vi "Run.vi"(8 "error in (no error)":errorcluster, 11 "Opctics in":refnum<class "Optics.lvclass">) -> (0 "error out":errorcluster, 3 "Optics out":refnum<class "Optics.lvclass">)   [LabVIEW 2018, in "Optics.lvclass"]
uses:
  Optics.lvclass
  Optics.lvclass/Optics.ctl
  Device.lvclass
  StateMachine/State Machine.lvclass
panel:
  out "on target 3":bool
  out "on target 2":bool
  out "on target":bool
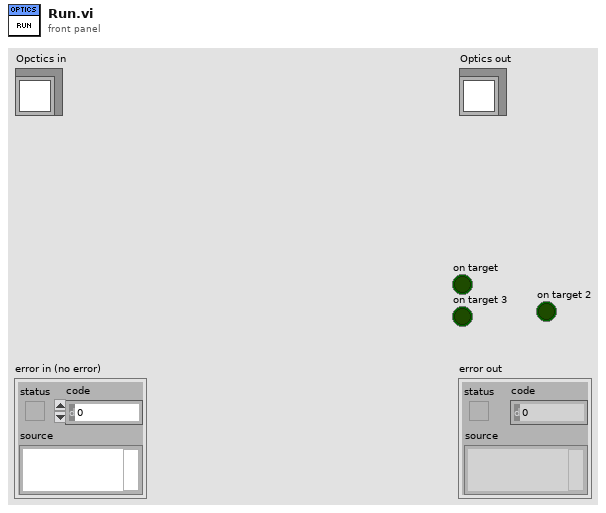
[diagram p1: front panel]
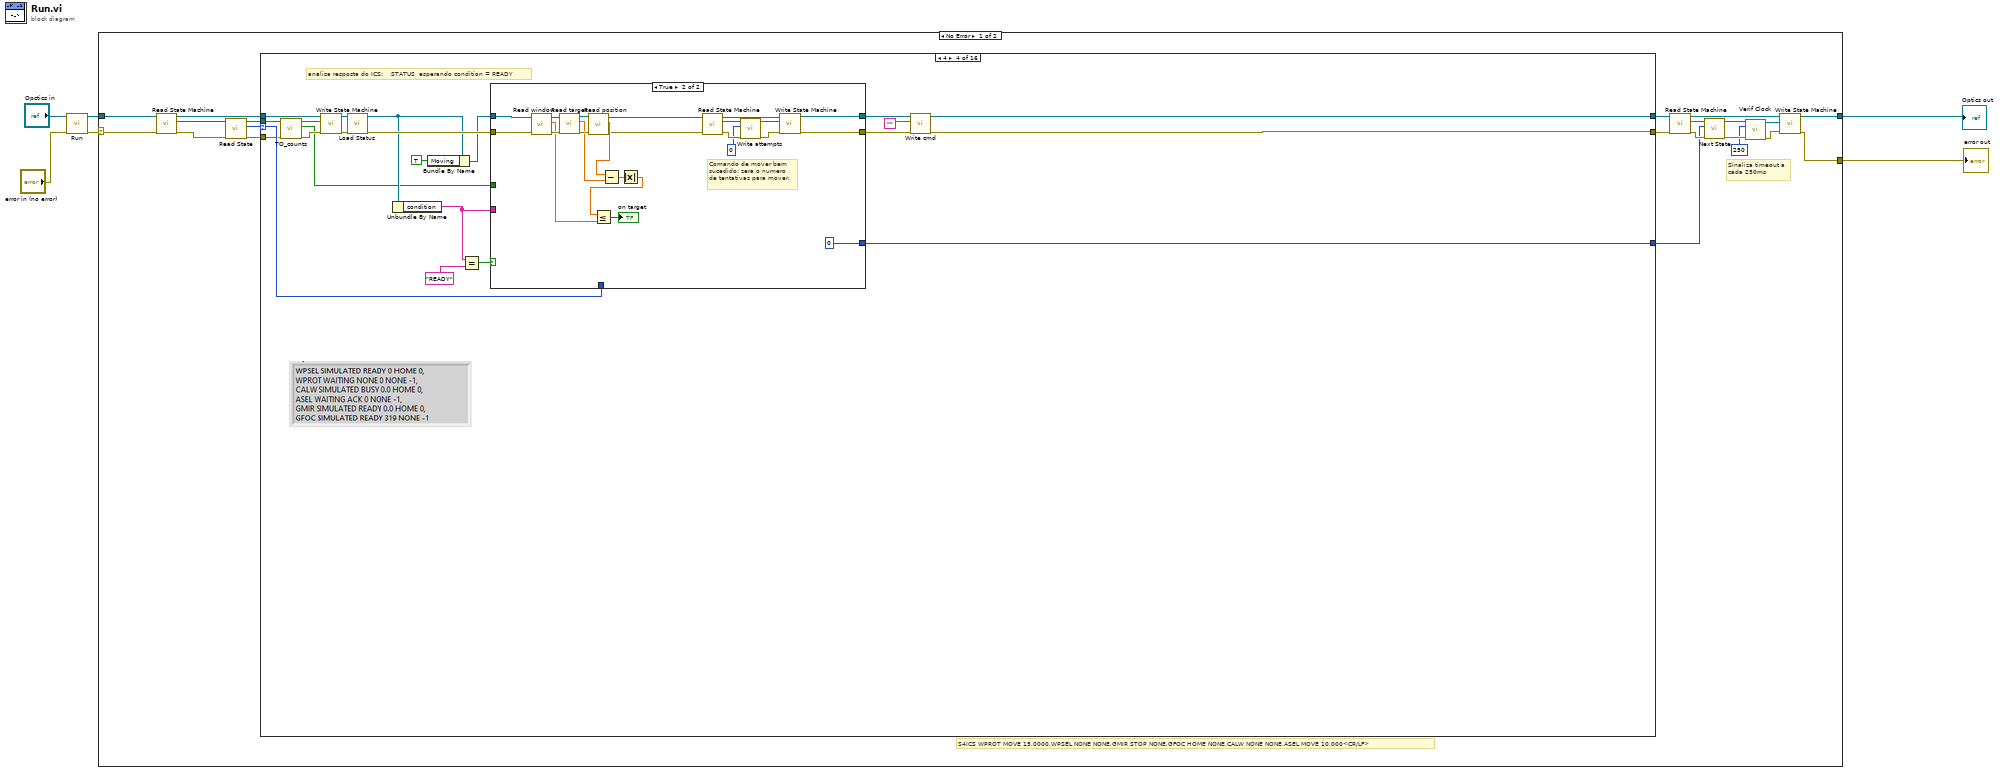
[diagram p0: block diagram]
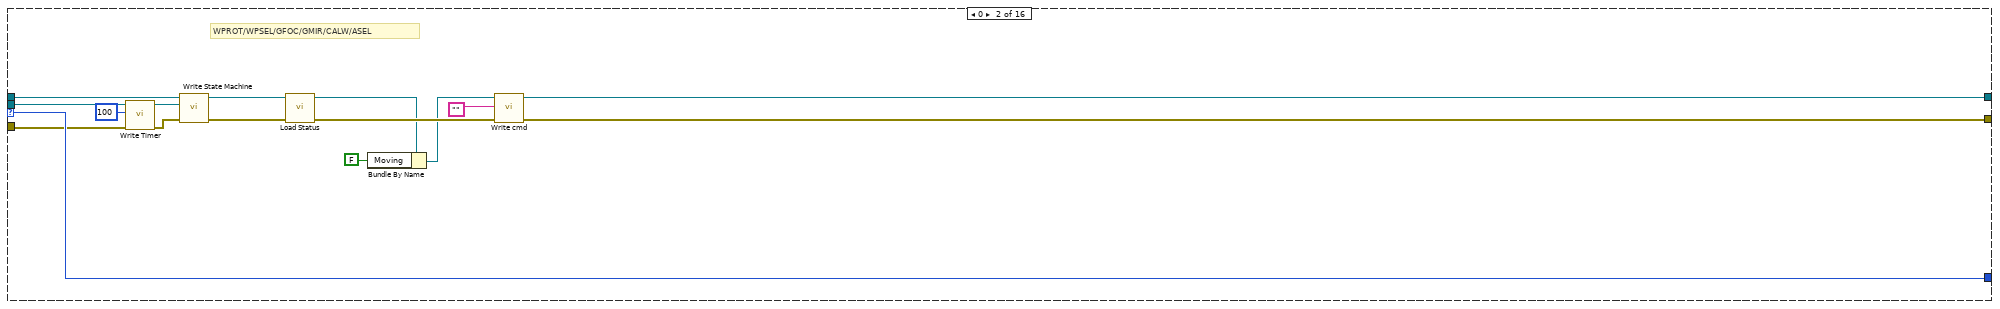
[diagram p3: hidden frame]
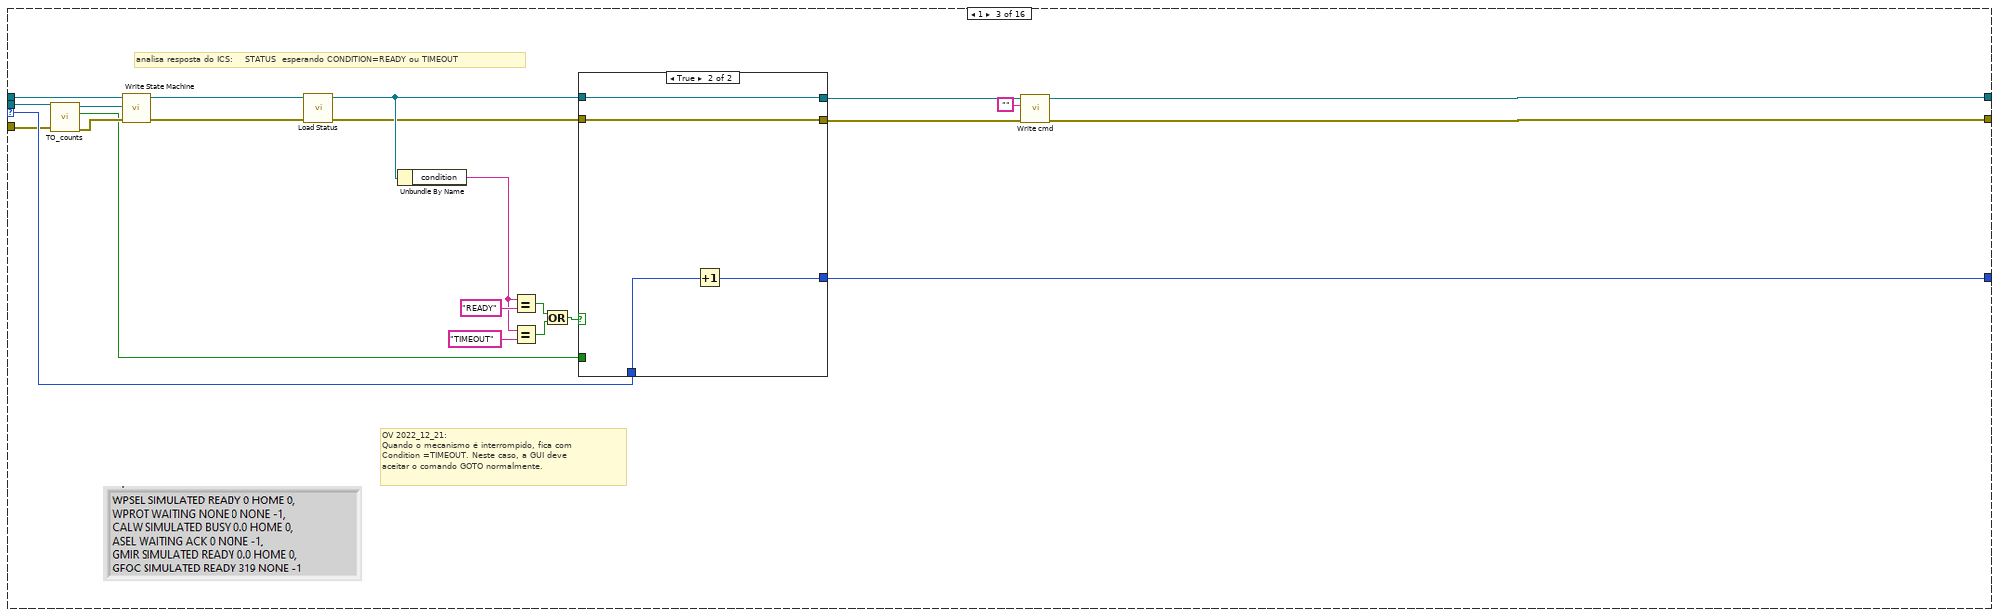
[diagram p4: hidden frame]
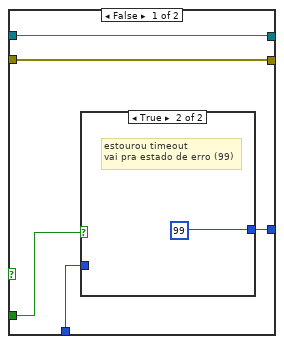
[diagram p5: hidden frame]
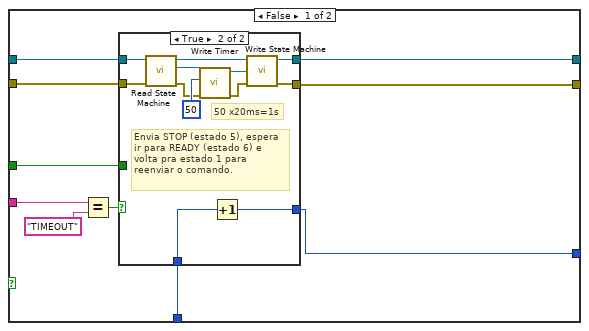
[diagram p7: hidden frame]
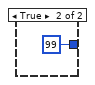
[diagram p9: hidden frame]
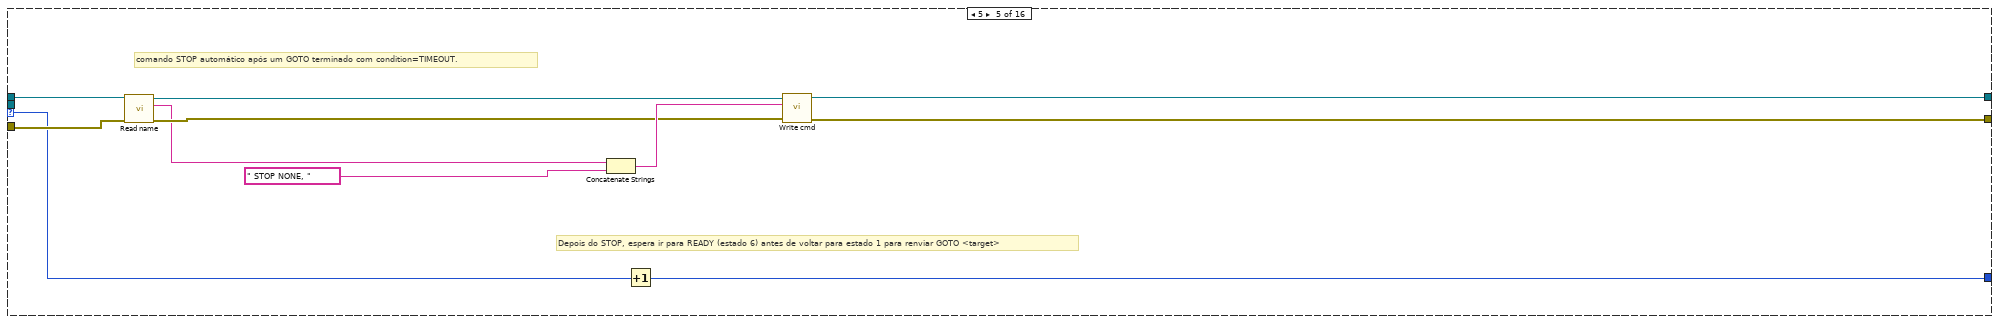
[diagram p10: hidden frame]
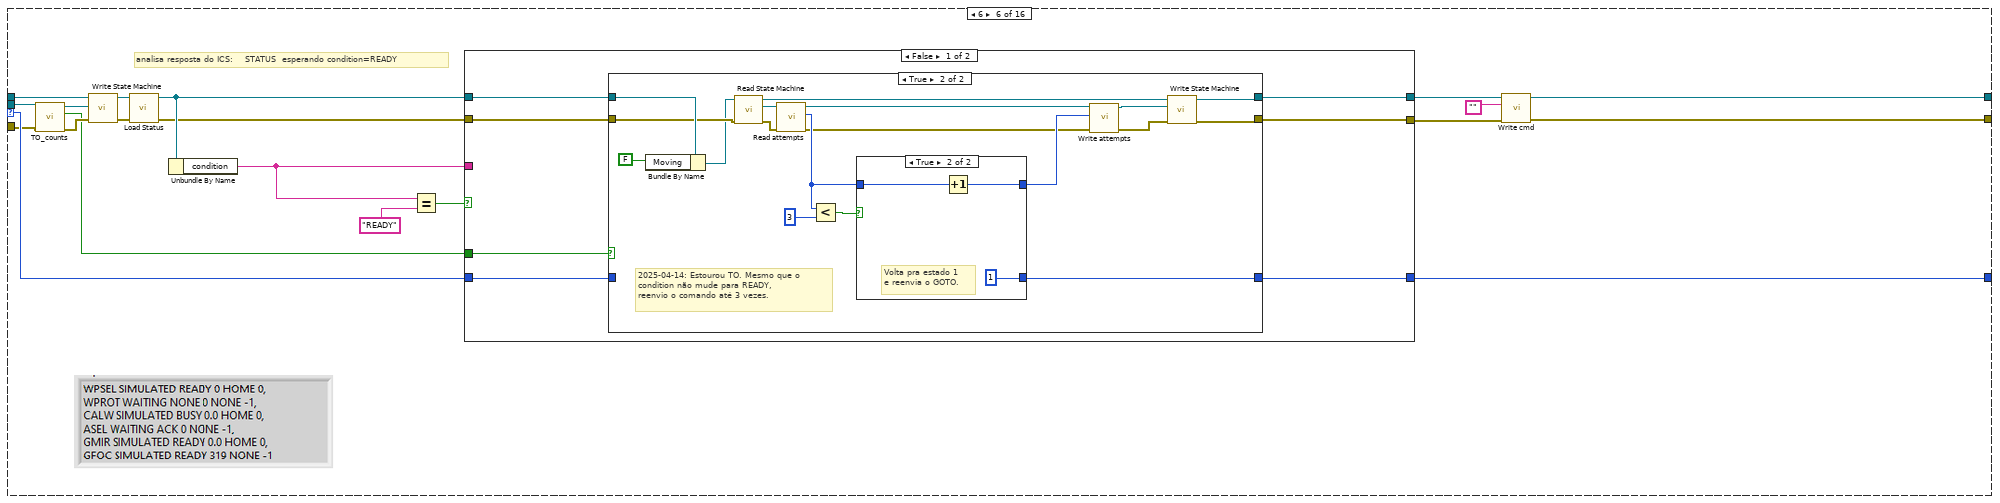
[diagram p11: hidden frame]
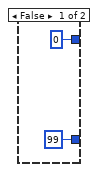
[diagram p13: hidden frame]
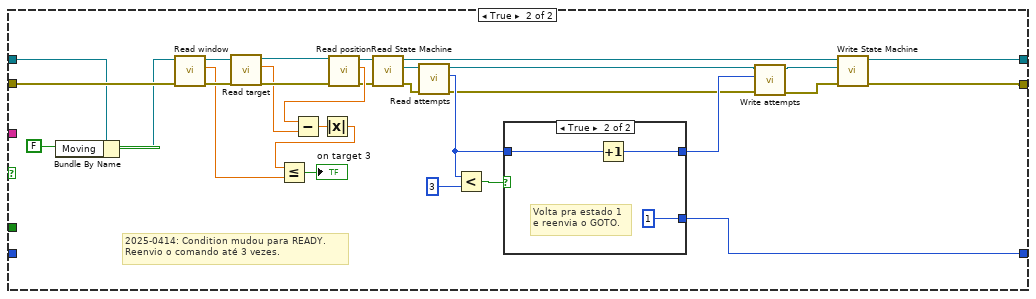
[diagram p14: hidden frame]
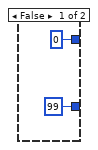
[diagram p15: hidden frame]
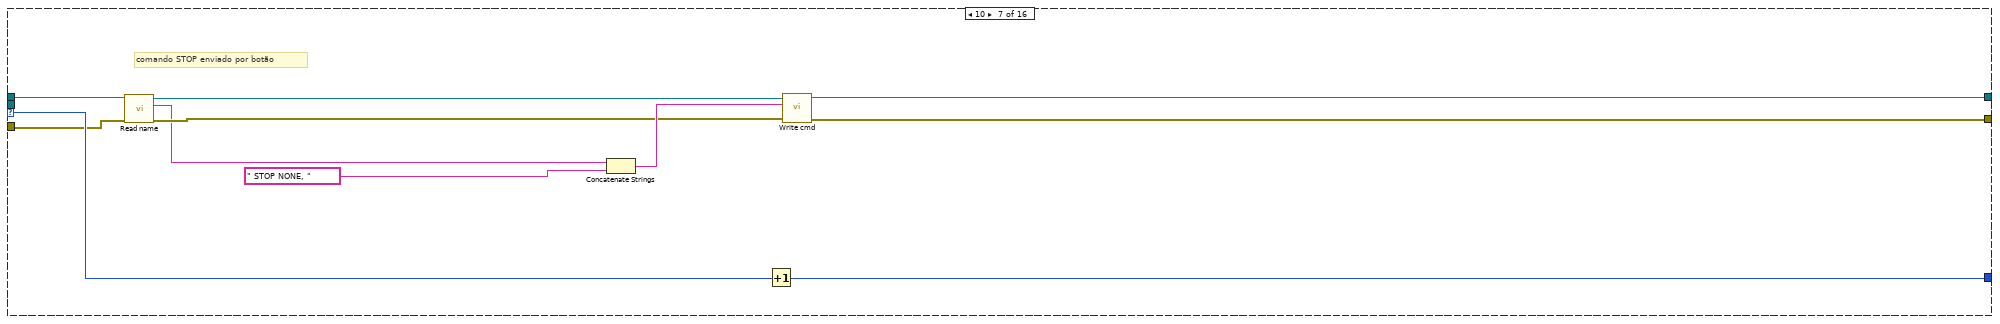
[diagram p16: hidden frame]
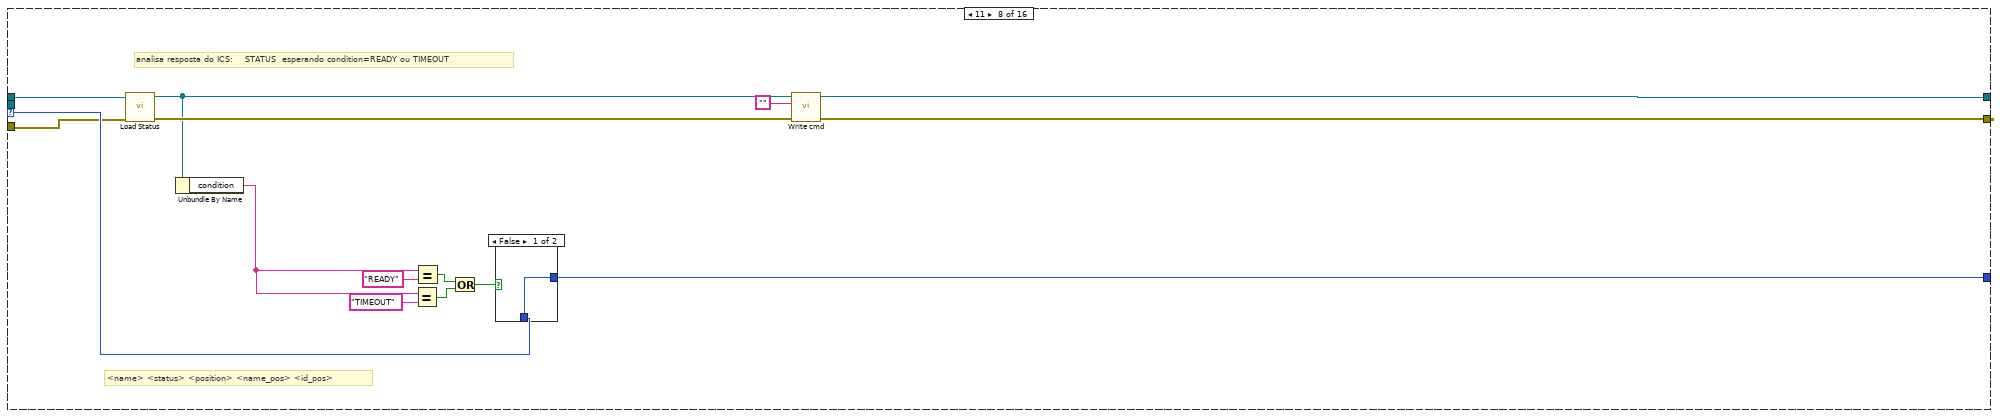
[diagram p17: hidden frame]
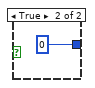
[diagram p18: hidden frame]
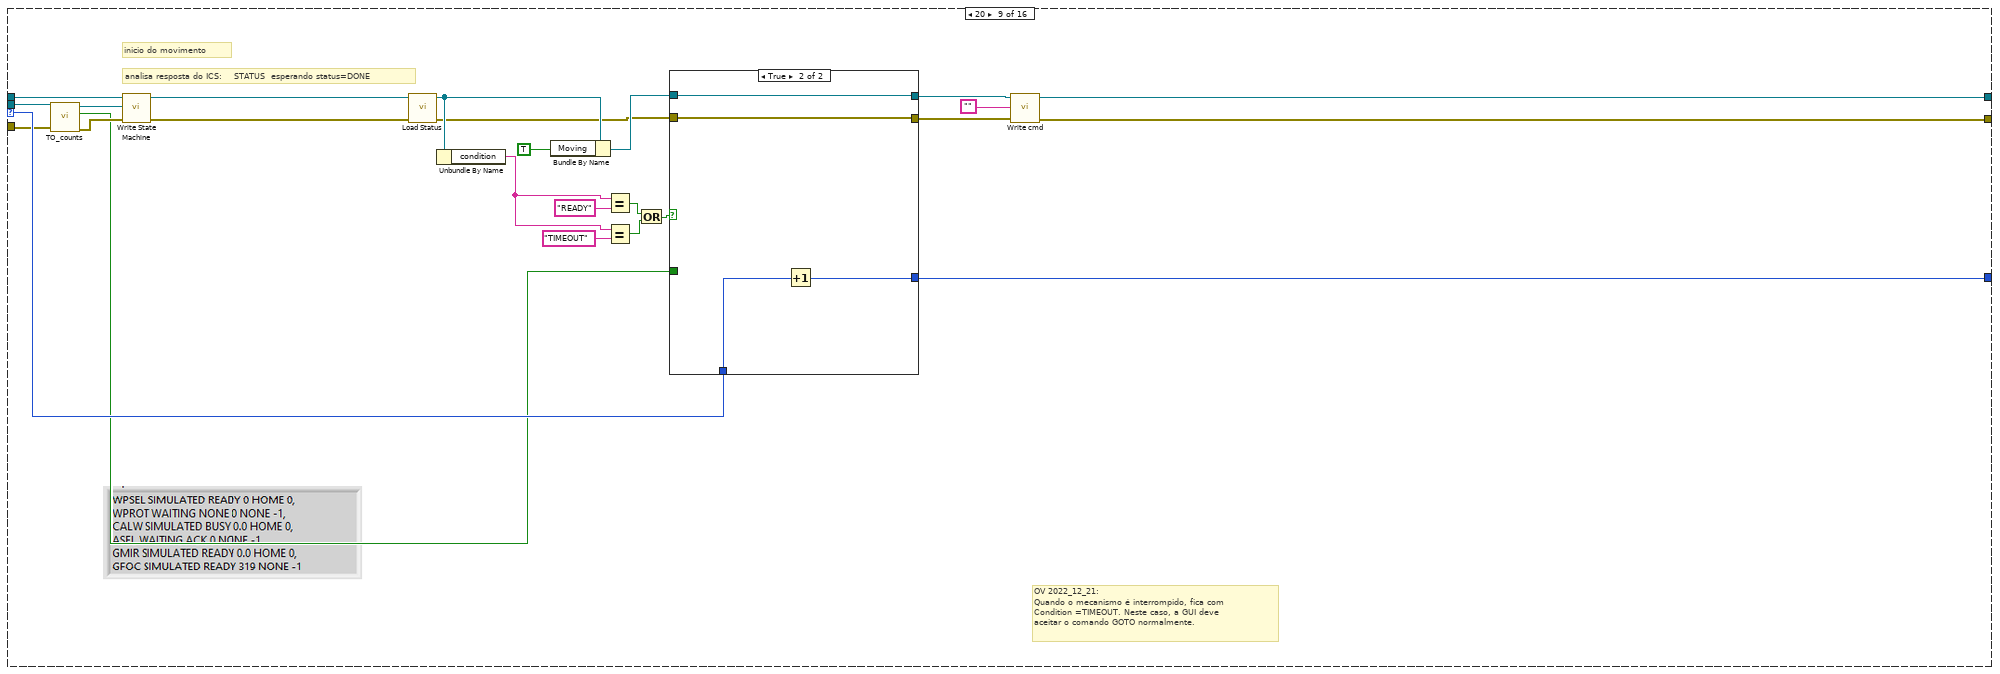
[diagram p19: hidden frame]
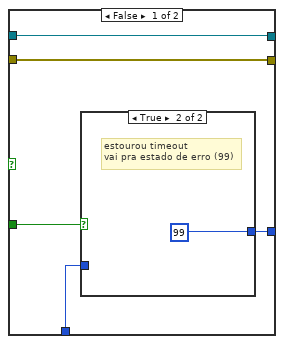
[diagram p20: hidden frame]
diagram:
  n1 = call-parent "Run.vi"("error in (no error)"="error in (no error)", "Device in"="Opctics in") -> ("error out"=w4:errorcluster, "Device out"=w3:refnum<class "Optics.lvclass">)  [unwired: 8 in]
  n2 = case shown="No Error" w4 {
    selector: w4 -> [w16 w465]
    tunnel: [w19 w465] -> w1
    tunnel: [w22 w464] -> w2
    tunnel: w3 -> [w17 w464]
    frame No Error {
      # "Sinaliza timeout a\ncada 250ms"
      # "S4ICS WPROT MOVE 15.0000,WPSEL NONE NONE,GMIR STOP NONE,GFOC HOME NONE,CALW NONE NONE,ASEL MOVE 10.000<CR/LF>"
      n3 = call-dynamic "Read State Machine.vi"("error in (no error)"=w16, "Device in"=w17) -> ("error out"=w15:errorcluster, "State Machine.lvclass"=w14:refnum<class "State Machine.lvclass">, "Device out"=w25:refnum<class "Optics.lvclass">)  [unwired: 7 in]
      n4 = call-dynamic "Read State.vi"("error in (no error)"=w15, "State Machine in"=w14) -> ("error out"=w26:errorcluster, "State"=w27:i32, "State Machine out"=w18:refnum<class "State Machine.lvclass">)  [unwired: 7 in]
      n5 = case shown="4" w27 {
        selector: w27 -> [w28 w43 w66 w99 w156 w182 w261 w279 w303 w331 w347 w381 w403 w422 w441 w461]
        tunnel: w26 -> [w29 w41 w62 w81 w159 w171 w256 w268 w299 w322 w340 w375 w395 w416 w434 w456]
        tunnel: [w29 w45 w68 w101 w164 w184 w263 w276 w305 w328 w349 w384 w400 w420 w438 w462] -> w8
        tunnel: w25 -> [w30 w42 w65 w85 w161 w169 w258 w269 w302 w323 w339 w374 w399 w423 w437 w457]
        tunnel: [w30 w46 w69 w102 w165 w185 w264 w277 w306 w329 w350 w385 w401 w421 w439 w463] -> w7
        tunnel: [w28 w43 w67 w100 w155 w183 w262 w278 w304 w330 w348 w382 w402 w419 w440 w461] -> w20
        tunnel: w18 -> [_ w39 w64 w86 _ w170 _ _ w301 _ _ w376 w397 w418 w436 _]
        frame Default {
        }
        frame 0 {
          # "WPROT/WPSEL/GFOC/GMIR/CALW/ASEL"
          n6 = call-dynamic "Write Timer.vi"("error in (no error)"=w41, "Timer"=u32 100, "State Machine in"=w39) -> ("error out"=w40:errorcluster, "State Machine out"=w38:refnum<class "State Machine.lvclass">)  [unwired: 7 in]
          n7 = call-dynamic "Write State Machine.vi"("error in (no error)"=w40, "State Machine.lvclass"=w38, "Device in"=w42) -> ("error out"=w35:errorcluster, "Device out"=w36:refnum<class "Optics.lvclass">)  [unwired: 7 in]
          n8 = call-dynamic "Load Status.vi"("error in (no error)"=w35, "Optics in"=w36) -> ("error out"=w34:errorcluster, "Optics out"=w33:refnum<class "Optics.lvclass">)  [unwired: 8 in]
          n9 = Bundle By Name(cluster=w33, "Moving"=FALSE) -> (w31:refnum<class "Optics.lvclass">)
          n10 = call-dynamic "Write cmd.vi"("error in (no error)"=w34, "cmd"="", "Device in"=w31) -> ("error out"=w45:errorcluster, "Device out"=w46:refnum<class "Optics.lvclass">)  [unwired: 7 in]
        }
        frame 1 {
          # "OV 2022_12_21:\nQuando o mecanismo é interrompido, fica com\nCondition =TIMEOUT. Neste caso, a GUI deve\naceitar o comando GOTO normalmente."
          # "analisa resposta do ICS:    STATUS  esperando CONDITION=READY ou TIMEOUT"
          n11 = call-dynamic "TO_counts.vi"("error in (no error)"=w62, "State Machine in"=w64) -> ("error out"=w61:errorcluster, "timer zero"=w60:bool, "State Machine out"=w63:refnum<class "State Machine.lvclass">)  [unwired: 7 in]
          n12 = call-dynamic "Write State Machine.vi"("error in (no error)"=w61, "State Machine.lvclass"=w63, "Device in"=w65) -> ("error out"=w50:errorcluster, "Device out"=w51:refnum<class "Optics.lvclass">)  [unwired: 7 in]
          n13 = call-dynamic "Load Status.vi"("error in (no error)"=w50, "Optics in"=w51) -> ("error out"=w48:errorcluster, "Optics out"=w49:refnum<class "Optics.lvclass">)  [unwired: 8 in]
          n14 = Unbundle By Name(w49) -> ("condition"=w47:string)
          n15 = Equal?(x=w47, y="READY") -> (x = y?=w53:bool)
          n16 = Equal?(x=w47, y="TIMEOUT") -> (x = y?=w52:bool)
          n17 = Or(x=w53, y=w52) -> (x .or. y?=w54:bool)
          n18 = case shown="True" w54 {
            tunnel: [w72 w77] -> w67
            tunnel: w66 -> [w71 w78]
            tunnel: w49 -> [w74 w80]
            tunnel: w48 -> [w73 w79]
            tunnel: [w74 w80] -> w58
            tunnel: [w73 w79] -> w59
            tunnel: w60 -> [w70 _]
            frame False {
              n19 = case shown="True" w70 {
                tunnel: [w75 99 ("State")] -> w72
                tunnel: w71 -> [w75 _]
                frame False {
                  # "Não estourou timeout"
                }
                frame True {
                  # "estourou timeout\nvai pra estado de erro (99)"
                }
              }
            }
            frame True {
              n20 = Increment(x=w78) -> (x+1=w77:i32)
            }
          }
          n21 = call-dynamic "Write cmd.vi"("error in (no error)"=w59, "cmd"="", "Device in"=w58) -> ("error out"=w68:errorcluster, "Device out"=w69:refnum<class "Optics.lvclass">)  [unwired: 7 in]
        }
        frame 4 {
          # "analisa resposta do ICS:    STATUS  esperando condition = READY"
          n22 = call-dynamic "TO_counts.vi"("error in (no error)"=w81, "State Machine in"=w86) -> ("error out"=w87:errorcluster, "timer zero"=w84:bool, "State Machine out"=w88:refnum<class "State Machine.lvclass">)  [unwired: 7 in]
          n23 = call-dynamic "Write State Machine.vi"("error in (no error)"=w87, "State Machine.lvclass"=w88, "Device in"=w85) -> ("error out"=w82:errorcluster, "Device out"=w83:refnum<class "Optics.lvclass">)  [unwired: 7 in]
          n24 = call-dynamic "Load Status.vi"("error in (no error)"=w82, "Optics in"=w83) -> ("error out"=w93:errorcluster, "Optics out"=w91:refnum<class "Optics.lvclass">)  [unwired: 8 in]
          n25 = Unbundle By Name(w91) -> ("condition"=w92:string)
          n26 = Bundle By Name(cluster=w91, "Moving"=TRUE) -> (w90:refnum<class "Optics.lvclass">)
          n27 = Equal?(x=w92, y="READY") -> (x = y?=w94:bool)
          n28 = case shown="True" w94 {
            tunnel: [w111 0 ("t")] -> w100
            tunnel: w99 -> [w112 _]
            tunnel: w90 -> [w107 w142]
            tunnel: w93 -> [w105 w147]
            tunnel: [w106 w139] -> w97
            tunnel: [w104 w135] -> w98
            tunnel: w92 -> [w108 _]
            tunnel: w84 -> [w103 _]
            frame False {
              n29 = Equal?(x=w108, y="TIMEOUT") -> (x = y?=w109:bool)
              n30 = case shown="True" w109 {
                tunnel: w112 -> [w115 w121]
                tunnel: [w114 w120] -> w111
                tunnel: w107 -> [w117 w131]
                tunnel: [w117 w126] -> w106
                tunnel: w105 -> [w116 w130]
                tunnel: [w116 w124] -> w104
                tunnel: w103 -> [w113 _]
                frame False {
                  n31 = case shown="False" w113 {
                    tunnel: [w118 99 ("State")] -> w114
                    tunnel: w115 -> [w118 _]
                    frame False {
                    }
                    frame True {
                    }
                  }
                }
                frame True {
                  # "50 x20ms=1s"
                  # "Envia STOP (estado 5), espera\nir para READY (estado 6) e\nvolta pra estado 1 para\nreenviar o comando."
                  n32 = call-dynamic "Read State Machine.vi"("error in (no error)"=w130, "Device in"=w131) -> ("error out"=w127:errorcluster, "State Machine.lvclass"=w129:refnum<class "State Machine.lvclass">, "Device out"=w122:refnum<class "Optics.lvclass">)  [unwired: 7 in]
                  n33 = call-dynamic "Write Timer.vi"("error in (no error)"=w127, "Timer"=u32 50, "State Machine in"=w129) -> ("error out"=w125:errorcluster, "State Machine out"=w123:refnum<class "State Machine.lvclass">)  [unwired: 7 in]
                  n34 = Increment(x=w121) -> (x+1=w120:i32)
                  n35 = call-dynamic "Write State Machine.vi"("error in (no error)"=w125, "State Machine.lvclass"=w123, "Device in"=w122) -> ("error out"=w124:errorcluster, "Device out"=w126:refnum<class "Optics.lvclass">)  [unwired: 7 in]
                }
              }
            }
            frame True {
              # "Comando de mover bem\nsucedido: zera o numero \nde tentativas para mover."
              n36 = call "Read window.vi"("error in (no error)"=w147, "Optics in"=w142) -> ("error out"=w146:errorcluster, "window"=w145:dbl, "Optics out"=w148:refnum<class "Optics.lvclass">)  [unwired: 7 in]
              n37 = call "Read target.vi"("error in (no error)"=w146, "Optics in"=w148) -> ("error out"=w154:errorcluster, "target"=w152:dbl, "Optics out"=w153:refnum<class "Optics.lvclass">)  [unwired: 7 in]
              n38 = call "Read position.vi"("error in (no error)"=w154, "Optics in"=w153) -> ("error out"=w138:errorcluster, "position"=w151:dbl, "Optics out"=w141:refnum<class "Optics.lvclass">)  [unwired: 7 in]
              n39 = Subtract(x=w151, y=w152) -> (x-y=w150:dbl)
              n40 = Absolute Value(x=w150) -> (abs(x)=w149:dbl)
              n41 = Less Or Equal?(x=w149, y=w145) -> (x <= y?=→"on target":bool)
              n42 = call-dynamic "Read State Machine.vi"("error in (no error)"=w138, "Device in"=w141) -> ("error out"=w134:errorcluster, "State Machine.lvclass"=w137:refnum<class "State Machine.lvclass">, "Device out"=w140:refnum<class "Optics.lvclass">)  [unwired: 7 in]
              n43 = call-dynamic "Write attempts.vi"("error in (no error)"=w134, "attempts"=u32 0, "State Machine in"=w137) -> ("error out"=w133:errorcluster, "State Machine out"=w136:refnum<class "State Machine.lvclass">)  [unwired: 7 in]
              n44 = call-dynamic "Write State Machine.vi"("error in (no error)"=w133, "State Machine.lvclass"=w136, "Device in"=w140) -> ("error out"=w135:errorcluster, "Device out"=w139:refnum<class "Optics.lvclass">)  [unwired: 7 in]
            }
          }
          n45 = call-dynamic "Write cmd.vi"("error in (no error)"=w98, "cmd"="", "Device in"=w97) -> ("error out"=w101:errorcluster, "Device out"=w102:refnum<class "Optics.lvclass">)  [unwired: 7 in]
        }
        frame 5 {
          # "Depois do STOP, espera ir para READY (estado 6) antes de voltar para estado 1 para renviar GOTO <target>"
          # "comando STOP automático após um GOTO terminado com condition=TIMEOUT."
          n46 = call "Read name.vi"("error in (no error)"=w159, "Optics in"=w161) -> ("error out"=w158:errorcluster, "name"=w157:string, "Optics out"=w160:refnum<class "Optics.lvclass">)  [unwired: 7 in]
          n47 = Concatenate Strings(w157, " STOP NONE, " ("string")) -> (w162:string)
          n48 = Increment(x=w156) -> (x+1=w155:i32)
          n49 = call-dynamic "Write cmd.vi"("error in (no error)"=w158, "cmd"=w162, "Device in"=w160) -> ("error out"=w164:errorcluster, "Device out"=w165:refnum<class "Optics.lvclass">)  [unwired: 7 in]
        }
        frame 6 {
          # "analisa resposta do ICS:    STATUS  esperando condition=READY"
          n50 = call-dynamic "TO_counts.vi"("error in (no error)"=w171, "State Machine in"=w170) -> ("error out"=w172:errorcluster, "timer zero"=w166:bool, "State Machine out"=w173:refnum<class "State Machine.lvclass">)  [unwired: 7 in]
          n51 = call-dynamic "Write State Machine.vi"("error in (no error)"=w172, "State Machine.lvclass"=w173, "Device in"=w169) -> ("error out"=w167:errorcluster, "Device out"=w168:refnum<class "Optics.lvclass">)  [unwired: 7 in]
          n52 = call-dynamic "Load Status.vi"("error in (no error)"=w167, "Optics in"=w168) -> ("error out"=w174:errorcluster, "Optics out"=w175:refnum<class "Optics.lvclass">)  [unwired: 8 in]
          n53 = Unbundle By Name(w175) -> ("condition"=w176:string)
          n54 = Equal?(x=w176, y="READY") -> (x = y?=w177:bool)
          n55 = case shown="False" w177 {
            tunnel: [w190 w237] -> w183
            tunnel: w182 -> [w191 _]
            tunnel: w175 -> [w189 w235]
            tunnel: w174 -> [w188 w241]
            tunnel: [w187 w219] -> w180
            tunnel: [w186 w220] -> w181
            tunnel: w176 -> [_ _]
            tunnel: w166 -> [w192 _]
            frame False {
              n56 = case shown="True" w192 {
                tunnel: [w195 w199] -> w190
                tunnel: w191 -> [w195 _]
                tunnel: [w194 w198] -> w187
                tunnel: w189 -> [w194 w202]
                tunnel: [w193 w197] -> w186
                tunnel: w188 -> [w193 w201]
                frame False {
                  # "Aguarda \"condition\" mudar para READY."
                }
                frame True {
                  # "2025-04-14: Estourou TO. Mesmo que o\ncondition não mude para READY,\nreenvio o comando até 3 vezes."
                  n57 = Bundle By Name(cluster=w202, "Moving"=FALSE) -> (w200:refnum<class "Optics.lvclass">)
                  n58 = call-dynamic "Read State Machine.vi"("error in (no error)"=w201, "Device in"=w200) -> ("error out"=w209:errorcluster, "State Machine.lvclass"=w210:refnum<class "State Machine.lvclass">, "Device out"=w213:refnum<class "Optics.lvclass">)  [unwired: 7 in]
                  n59 = call-dynamic "Read attempts.vi"("error in (no error)"=w209, "State Machine in"=w210) -> ("error out"=w203:errorcluster, "attempts"=w206:u32, "State Machine out"=w204:refnum<class "State Machine.lvclass">)  [unwired: 7 in]
                  n60 = Less?(x=w206, y=u32 3) -> (x < y?=w207:bool)
                  n61 = case shown="True" w207 {
                    tunnel: [99 ("t") 1 ("t")] -> w199
                    tunnel: [u32 0 w216] -> w205
                    tunnel: w206 -> [_ w217]
                    frame False {
                    }
                    frame True {
                      # "Volta pra estado 1 \ne reenvia o GOTO."
                      n62 = Increment(x=w217) -> (x+1=w216:u32)
                    }
                  }
                  n63 = call-dynamic "Write attempts.vi"("error in (no error)"=w203, "attempts"=w205, "State Machine in"=w204) -> ("error out"=w212:errorcluster, "State Machine out"=w211:refnum<class "State Machine.lvclass">)  [unwired: 7 in]
                  n64 = call-dynamic "Write State Machine.vi"("error in (no error)"=w212, "State Machine.lvclass"=w211, "Device in"=w213) -> ("error out"=w197:errorcluster, "Device out"=w198:refnum<class "Optics.lvclass">)  [unwired: 7 in]
                }
              }
            }
            frame True {
              # "2025-0414: Condition mudou para READY.\nReenvio o comando até 3 vezes."
              n65 = Bundle By Name(cluster=w235, "Moving"=FALSE) -> (w234:refnum<class "Optics.lvclass">)
              n66 = call "Read window.vi"("error in (no error)"=w241, "Optics in"=w234) -> ("error out"=w240:errorcluster, "window"=w239:dbl, "Optics out"=w242:refnum<class "Optics.lvclass">)  [unwired: 7 in]
              n67 = call "Read target.vi"("error in (no error)"=w240, "Optics in"=w242) -> ("error out"=w248:errorcluster, "target"=w246:dbl, "Optics out"=w247:refnum<class "Optics.lvclass">)  [unwired: 7 in]
              n68 = call "Read position.vi"("error in (no error)"=w248, "Optics in"=w247) -> ("error out"=w227:errorcluster, "position"=w245:dbl, "Optics out"=w228:refnum<class "Optics.lvclass">)  [unwired: 7 in]
              n69 = Subtract(x=w245, y=w246) -> (x-y=w244:dbl)
              n70 = Absolute Value(x=w244) -> (abs(x)=w243:dbl)
              n71 = Less Or Equal?(x=w243, y=w239) -> (x <= y?=→"on target 3":bool)
              n72 = call-dynamic "Read State Machine.vi"("error in (no error)"=w227, "Device in"=w228) -> ("error out"=w229:errorcluster, "State Machine.lvclass"=w230:refnum<class "State Machine.lvclass">, "Device out"=w233:refnum<class "Optics.lvclass">)  [unwired: 7 in]
              n73 = call-dynamic "Read attempts.vi"("error in (no error)"=w229, "State Machine in"=w230) -> ("error out"=w221:errorcluster, "attempts"=w224:u32, "State Machine out"=w222:refnum<class "State Machine.lvclass">)  [unwired: 7 in]
              n74 = Less?(x=w224, y=u32 3) -> (x < y?=w225:bool)
              n75 = case shown="True" w225 {
                tunnel: [99 ("t") 1 ("t")] -> w237
                tunnel: [u32 0 w251] -> w223
                tunnel: w224 -> [_ w252]
                frame False {
                }
                frame True {
                  # "Volta pra estado 1 \ne reenvia o GOTO."
                  n76 = Increment(x=w252) -> (x+1=w251:u32)
                }
              }
              n77 = call-dynamic "Write attempts.vi"("error in (no error)"=w221, "attempts"=w223, "State Machine in"=w222) -> ("error out"=w232:errorcluster, "State Machine out"=w231:refnum<class "State Machine.lvclass">)  [unwired: 7 in]
              n78 = call-dynamic "Write State Machine.vi"("error in (no error)"=w232, "State Machine.lvclass"=w231, "Device in"=w233) -> ("error out"=w220:errorcluster, "Device out"=w219:refnum<class "Optics.lvclass">)  [unwired: 7 in]
            }
          }
          n79 = call-dynamic "Write cmd.vi"("error in (no error)"=w181, "cmd"="", "Device in"=w180) -> ("error out"=w184:errorcluster, "Device out"=w185:refnum<class "Optics.lvclass">)  [unwired: 7 in]
        }
        frame 10 {
          # "comando STOP enviado por botão"
          n80 = call "Read name.vi"("error in (no error)"=w256, "Optics in"=w258) -> ("error out"=w255:errorcluster, "name"=w254:string, "Optics out"=w257:refnum<class "Optics.lvclass">)  [unwired: 7 in]
          n81 = Concatenate Strings(w254, " STOP NONE, " ("string")) -> (w259:string)
          n82 = Increment(x=w261) -> (x+1=w262:i32)
          n83 = call-dynamic "Write cmd.vi"("error in (no error)"=w255, "cmd"=w259, "Device in"=w257) -> ("error out"=w263:errorcluster, "Device out"=w264:refnum<class "Optics.lvclass">)  [unwired: 7 in]
        }
        frame 11 {
          # "<name> <status> <position> <name_pos> <id_pos>"
          # "analisa resposta do ICS:    STATUS  esperando condition=READY ou TIMEOUT"
          n84 = call-dynamic "Load Status.vi"("error in (no error)"=w268, "Optics in"=w269) -> ("error out"=w266:errorcluster, "Optics out"=w265:refnum<class "Optics.lvclass">)  [unwired: 8 in]
          n85 = Unbundle By Name(w265) -> ("condition"=w267:string)
          n86 = Equal?(x=w267, y="TIMEOUT") -> (x = y?=w271:bool)
          n87 = Equal?(x=w267, y="READY") -> (x = y?=w272:bool)
          n88 = Or(x=w272, y=w271) -> (x .or. y?=w270:bool)
          n89 = case shown="False" w270 {
            tunnel: [w280 0] -> w278
            tunnel: w279 -> [w280 _]
            frame False {
            }
            frame True {
            }
          }
          n90 = call-dynamic "Write cmd.vi"("error in (no error)"=w266, "cmd"="", "Device in"=w265) -> ("error out"=w276:errorcluster, "Device out"=w277:refnum<class "Optics.lvclass">)  [unwired: 7 in]
        }
        frame 20 {
          # "OV 2022_12_21:\nQuando o mecanismo é interrompido, fica com\nCondition =TIMEOUT. Neste caso, a GUI deve\naceitar o comando GOTO normalmente."
          # "inicio do movimento"
          # "analisa resposta do ICS:    STATUS  esperando status=DONE"
          n91 = call-dynamic "TO_counts.vi"("error in (no error)"=w299, "State Machine in"=w301) -> ("error out"=w298:errorcluster, "timer zero"=w297:bool, "State Machine out"=w300:refnum<class "State Machine.lvclass">)  [unwired: 7 in]
          n92 = call-dynamic "Write State Machine.vi"("error in (no error)"=w298, "State Machine.lvclass"=w300, "Device in"=w302) -> ("error out"=w286:errorcluster, "Device out"=w287:refnum<class "Optics.lvclass">)  [unwired: 7 in]
          n93 = call-dynamic "Load Status.vi"("error in (no error)"=w286, "Optics in"=w287) -> ("error out"=w282:errorcluster, "Optics out"=w284:refnum<class "Optics.lvclass">)  [unwired: 8 in]
          n94 = Unbundle By Name(w284) -> ("condition"=w285:string)
          n95 = Bundle By Name(cluster=w284, "Moving"=TRUE) -> (w283:refnum<class "Optics.lvclass">)
          n96 = Equal?(x=w285, y="READY") -> (x = y?=w289:bool)
          n97 = Equal?(x=w285, y="TIMEOUT") -> (x = y?=w288:bool)
          n98 = Or(x=w289, y=w288) -> (x .or. y?=w290:bool)
          n99 = case shown="True" w290 {
            tunnel: [w309 w314] -> w304
            tunnel: w303 -> [w308 w315]
            tunnel: w283 -> [w311 w317]
            tunnel: w282 -> [w310 w316]
            tunnel: [w311 w317] -> w294
            tunnel: [w310 w316] -> w295
            tunnel: w297 -> [w307 _]
            frame False {
              n100 = case shown="True" w307 {
                tunnel: [w312 99 ("State")] -> w309
                tunnel: w308 -> [w312 _]
                frame False {
                  # "Não estourou timeout"
                }
                frame True {
                  # "estourou timeout\nvai pra estado de erro (99)"
                }
              }
            }
            frame True {
              n101 = Increment(x=w315) -> (x+1=w314:i32)
            }
          }
          n102 = call-dynamic "Write cmd.vi"("error in (no error)"=w295, "cmd"="", "Device in"=w294) -> ("error out"=w305:errorcluster, "Device out"=w306:refnum<class "Optics.lvclass">)  [unwired: 7 in]
        }
        frame 22 {
          # "<SUBSYSTEM> <MODE> <CONDITION> <VALUE> <POSNAME> <POSID>"
          # "analisa resposta do ICS:    STATUS  esperando condition=BUSY"
          n103 = call-dynamic "Load Status.vi"("error in (no error)"=w322, "Optics in"=w323) -> ("error out"=w318:errorcluster, "Optics out"=w320:refnum<class "Optics.lvclass">)  [unwired: 8 in]
          n104 = Unbundle By Name(w320) -> ("condition"=w321:string)
          n105 = Equal?(x=w321, y="BUSY") -> (x = y?=w324:bool)
          n106 = Bundle By Name(cluster=w320, "Moving"=FALSE) -> (w319:refnum<class "Optics.lvclass">)
          n107 = case shown="True" w324 {
            tunnel: [w332 w333] -> w330
            tunnel: w331 -> [w332 w334]
            frame False {
            }
            frame True {
              n108 = Increment(x=w334) -> (x+1=w333:i32)
            }
          }
          n109 = call-dynamic "Write cmd.vi"("error in (no error)"=w318, "cmd"="", "Device in"=w319) -> ("error out"=w328:errorcluster, "Device out"=w329:refnum<class "Optics.lvclass">)  [unwired: 7 in]
        }
        frame 23 {
          # "analisa resposta do ICS:    STATUS  esperando condition <> BUSY"
          n110 = call-dynamic "Load Status.vi"("error in (no error)"=w340, "Optics in"=w339) -> ("error out"=w335:errorcluster, "Optics out"=w337:refnum<class "Optics.lvclass">)  [unwired: 8 in]
          n111 = Unbundle By Name(w337) -> ("condition"=w338:string)
          n112 = Bundle By Name(cluster=w337, "Moving"=TRUE) -> (w336:refnum<class "Optics.lvclass">)
          n113 = Not Equal?(x=w338, y="BUSY") -> (x != y?=w342:bool)
          n114 = case shown="True" w342 {
            tunnel: [w353 21 ("t")] -> w348
            tunnel: w347 -> [w353 _]
            tunnel: w336 -> [w352 w360]
            tunnel: w335 -> [w351 w358]
            tunnel: [w352 w366] -> w345
            tunnel: [w351 w365] -> w344
            frame False {
            }
            frame True {
              # "Repete o ciclo de\nmovimento continuo."
              n115 = call "Read window.vi"("error in (no error)"=w358, "Optics in"=w360) -> ("error out"=w357:errorcluster, "window"=w356:dbl, "Optics out"=w359:refnum<class "Optics.lvclass">)  [unwired: 7 in]
              n116 = call "Read target.vi"("error in (no error)"=w357, "Optics in"=w359) -> ("error out"=w368:errorcluster, "target"=w364:dbl, "Optics out"=w367:refnum<class "Optics.lvclass">)  [unwired: 7 in]
              n117 = call "Read position.vi"("error in (no error)"=w368, "Optics in"=w367) -> ("error out"=w365:errorcluster, "position"=w363:dbl, "Optics out"=w366:refnum<class "Optics.lvclass">)  [unwired: 7 in]
              n118 = Subtract(x=w363, y=w364) -> (x-y=w362:dbl)
              n119 = Absolute Value(x=w362) -> (abs(x)=w361:dbl)
              n120 = Less Or Equal?(x=w361, y=w356) -> (x <= y?=→"on target 2":bool)
            }
          }
          n121 = call-dynamic "Write cmd.vi"("error in (no error)"=w344, "cmd"="", "Device in"=w345) -> ("error out"=w349:errorcluster, "Device out"=w350:refnum<class "Optics.lvclass">)  [unwired: 7 in]
        }
        frame 30 {
          # "240 x 0,25s = 1min \npara completar homing"
          # "S4ICS GMIR INIT NONE"
          # "WPROT/WPSEL/GFOC/GMIR/CALW/ASEL"
          # "comando INIT"
          n122 = call-dynamic "Write Timer.vi"("error in (no error)"=w375, "Timer"=u32 240, "State Machine in"=w376) -> ("error out"=w371:errorcluster, "State Machine out"=w370:refnum<class "State Machine.lvclass">)  [unwired: 7 in]
          n123 = call-dynamic "Write State Machine.vi"("error in (no error)"=w371, "State Machine.lvclass"=w370, "Device in"=w374) -> ("error out"=w372:errorcluster, "Device out"=w373:refnum<class "Optics.lvclass">)  [unwired: 7 in]
          n124 = call "Read name.vi"("error in (no error)"=w372, "Optics in"=w373) -> ("error out"=w379:errorcluster, "name"=w377:string, "Optics out"=w378:refnum<class "Optics.lvclass">)  [unwired: 7 in]
          n125 = Concatenate Strings(w377, " INIT NONE, " ("string")) -> (w383:string)
          n126 = Increment(x=w381) -> (x+1=w382:i32)
          n127 = call-dynamic "Write cmd.vi"("error in (no error)"=w379, "cmd"=w383, "Device in"=w378) -> ("error out"=w384:errorcluster, "Device out"=w385:refnum<class "Optics.lvclass">)  [unwired: 7 in]
        }
        frame 31 {
          # "Timeout controlado\npor Verif Clock.vi"
          # "<name> <status> <position> <name_pos> <id_pos>"
          # "analisa resposta do ICS:    STATUS  esperando condition=BUSY"
          n128 = call-dynamic "Read Timeout.vi"("error in (no error)"=w395, "State Machine in"=w397) -> ("error out"=w394:errorcluster, "Timeout"=w393:bool, "State Machine out"=w396:refnum<class "State Machine.lvclass">)  [unwired: 7 in]
          n129 = call-dynamic "Write State Machine.vi"("error in (no error)"=w394, "State Machine.lvclass"=w396, "Device in"=w399) -> ("error out"=w389:errorcluster, "Device out"=w390:refnum<class "Optics.lvclass">)  [unwired: 7 in]
          n130 = call-dynamic "Load Status.vi"("error in (no error)"=w389, "Optics in"=w390) -> ("error out"=w387:errorcluster, "Optics out"=w386:refnum<class "Optics.lvclass">)  [unwired: 8 in]
          n131 = Unbundle By Name(w386) -> ("condition"=w388:string)
          n132 = Equal?(x=w388, y="BUSY") -> (x = y?=w392:bool)
          n133 = case shown="True" w392 {
            tunnel: [w405 w412] -> w402
            tunnel: w403 -> [w406 w413]
            tunnel: w393 -> [w404 _]
            frame False {
              n134 = case shown="True" w404 {
                tunnel: [w407 w409] -> w405
                tunnel: w406 -> [w407 w408]
                frame False {
                }
                frame True {
                  n135 = disable-structure shown="Enabled" {
                    disable-tunnel: [99 ("State") w411] -> w409
                    disable-tunnel: w408 -> [_ w411]
                    frame Disabled {
                    }
                    frame Enabled {
                    }
                  }
                }
              }
            }
            frame True {
              n136 = Increment(x=w413) -> (x+1=w412:i32)
            }
          }
          n137 = call-dynamic "Write cmd.vi"("error in (no error)"=w387, "cmd"="", "Device in"=w386) -> ("error out"=w400:errorcluster, "Device out"=w401:refnum<class "Optics.lvclass">)  [unwired: 7 in]
        }
        frame 32 {
          # "<name> <status> <position> <name_pos> <id_pos>"
          # "timeout  para terminar o movimento: 240 x 0,25s = 1 min"
          n138 = call-dynamic "Write Timer.vi"("error in (no error)"=w416, "Timer"=u32 240, "State Machine in"=w418) -> ("error out"=w415:errorcluster, "State Machine out"=w417:refnum<class "State Machine.lvclass">)  [unwired: 7 in]
          n139 = Increment(x=w422) -> (x+1=w419:i32)
          n140 = call-dynamic "Write State Machine.vi"("error in (no error)"=w415, "State Machine.lvclass"=w417, "Device in"=w423) -> ("error out"=w420:errorcluster, "Device out"=w421:refnum<class "Optics.lvclass">)  [unwired: 7 in]
        }
        frame 33 {
          # "<name> <status> <position> <name_pos> <id_pos>"
          # "analisa resposta do ICS:    STATUS  esperando condition <> BUSY"
          n141 = call-dynamic "TO_counts.vi"("error in (no error)"=w434, "State Machine in"=w436) -> ("error out"=w433:errorcluster, "timer zero"=w432:bool, "State Machine out"=w435:refnum<class "State Machine.lvclass">)  [unwired: 7 in]
          n142 = call-dynamic "Write State Machine.vi"("error in (no error)"=w433, "State Machine.lvclass"=w435, "Device in"=w437) -> ("error out"=w427:errorcluster, "Device out"=w428:refnum<class "Optics.lvclass">)  [unwired: 7 in]
          n143 = call-dynamic "Load Status.vi"("error in (no error)"=w427, "Optics in"=w428) -> ("error out"=w425:errorcluster, "Optics out"=w424:refnum<class "Optics.lvclass">)  [unwired: 8 in]
          n144 = Unbundle By Name(w424) -> ("condition"=w426:string)
          n145 = Not Equal?(x=w426, y="BUSY") -> (x != y?=w429:bool)
          n146 = case shown="True" w429 {
            tunnel: [w443 w453] -> w440
            tunnel: w441 -> [w444 _]
            tunnel: w432 -> [w442 _]
            tunnel: w426 -> [_ w451]
            frame False {
              n147 = case shown="False" w442 {
                tunnel: [w445 w447] -> w443
                tunnel: w444 -> [w445 w446]
                frame False {
                }
                frame True {
                  n148 = disable-structure shown="Disabled" {
                    disable-tunnel: [99 ("State") w449] -> w447
                    disable-tunnel: w446 -> [_ w449]
                    frame Disabled {
                    }
                    frame Enabled {
                    }
                  }
                }
              }
            }
            frame True {
              n149 = Equal?(x="READY" ("y"), y=w451) -> (x = y?=w455:bool)
              n150 = Select(t=0, s=w455, f=30) -> (s? t:f=w453:i32)
            }
          }
          n151 = call-dynamic "Write cmd.vi"("error in (no error)"=w425, "cmd"="", "Device in"=w424) -> ("error out"=w438:errorcluster, "Device out"=w439:refnum<class "Optics.lvclass">)  [unwired: 7 in]
        }
        frame 99 {
          # "WPROT/WPSEL/GFOC/GMIR/CALW/ASEL"
          n152 = call-dynamic "Load Status.vi"("error in (no error)"=w456, "Optics in"=w457) -> ("error out"=w458:errorcluster, "Optics out"=w459:refnum<class "Optics.lvclass">)  [unwired: 8 in]
          n153 = call-dynamic "Write cmd.vi"("error in (no error)"=w458, "cmd"="", "Device in"=w459) -> ("error out"=w462:errorcluster, "Device out"=w463:refnum<class "Optics.lvclass">)  [unwired: 7 in]
        }
      }
      n154 = call-dynamic "Read State Machine.vi"("error in (no error)"=w8, "Device in"=w7) -> ("error out"=w21:errorcluster, "State Machine.lvclass"=w24:refnum<class "State Machine.lvclass">, "Device out"=w23:refnum<class "Optics.lvclass">)  [unwired: 7 in]
      n155 = call "Next State.vi"("error in (no error)"=w21, "New_State"=w20, "State Machine in"=w24) -> ("error out"=w13:errorcluster, "State Machine out"=w11:refnum<class "State Machine.lvclass">)  [unwired: 7 in]
      n156 = call-dynamic "Verif Clock.vi"("error in (no error)"=w13, "period (ms)"=u32 250 ("period"), "State Machine in"=w11) -> ("error out"=w12:errorcluster, "State Machine out"=w10:refnum<class "State Machine.lvclass">)  [unwired: 6 in, 1 out]
      n157 = call-dynamic "Write State Machine.vi"("error in (no error)"=w12, "State Machine.lvclass"=w10, "Device in"=w23) -> ("error out"=w19:errorcluster, "Device out"=w22:refnum<class "Optics.lvclass">)  [unwired: 7 in]
    }
    frame Error {
    }
  }
  "error out" <- w1
  "Optics out" <- w2
